vi "Release-user-events.vi"(8 "error in (no error)":errorcluster, 11 "Object ref in":T1) -> (0 "error out":errorcluster, 3 "Object ref out":T1)   [LabVIEW 2013, in "SLMControl.lvlib" / "SC-Main.lvclass"]
uses:
  SC-Main.lvclass
  Object-reference.ctl
  SC-Main.lvclass/SC-Main.ctl
  Read Activity log.vi
  Read Error log.vi
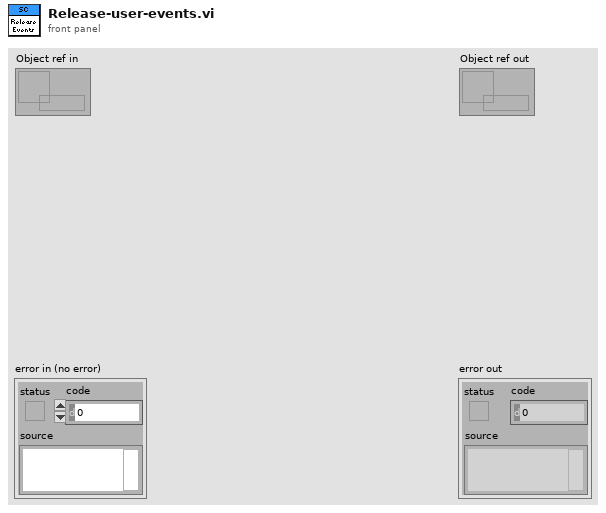
[diagram p1: front panel]
types:
  T1 = typedef "SLMControl.lvlib/SC-Main.lvclass/Object-reference.ctl" = refnum<data-value>
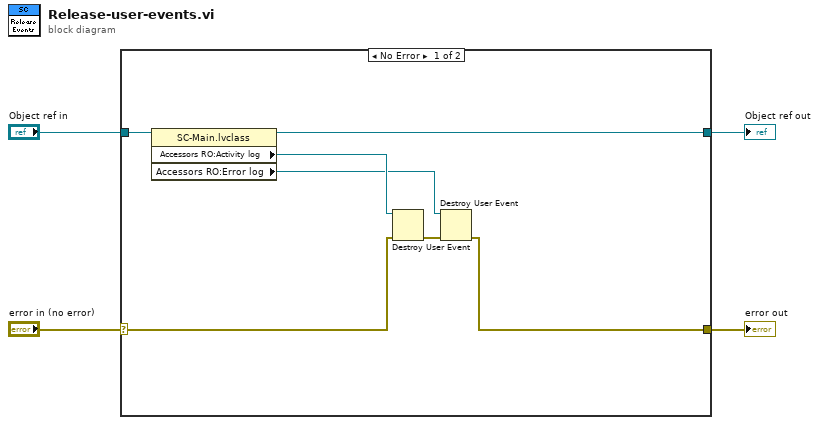
[diagram p0: block diagram]
diagram:
  n1 = case shown="No Error" "error in (no error)" {
    selector: "error in (no error)" -> [w5 w13]
    tunnel: [w7 w13] -> w3
    tunnel: [w10 w12] -> w1
    tunnel: "Object ref in" -> [w11 w12]
    frame No Error {
      n2 = property class="SC-Main.lvclass"(reference=w11) -> (reference out=w10:T1, "Accessors RO:Activity log"=w9:refnum<user-event>, "Accessors RO:Error log"=w6:refnum<user-event>)  [unwired: 1 in, 1 out]
      n3 = Destroy User Event(user event=w9, error in=w5) -> (error out=w8:errorcluster)
      n4 = Destroy User Event(user event=w6, error in=w8) -> (error out=w7:errorcluster)
    }
    frame Error {
    }
  }
  "error out" <- w3
  "Object ref out" <- w1
